vi "Owning System.vi"(8 "error in (no error)":errorcluster, 11 "Group in":refnum<class "Group.lvclass">) -> (0 "error out":errorcluster, 2 "Owning System":string, 3 "Group out":refnum<class "Group.lvclass">)   [LabVIEW 2020, in "VolatusConfig.lvlib" / "Group.lvclass"]
uses:
  Group.lvclass
  Group.lvclass/Group.ctl
  lv-cdm/CDM-Config/Config Manager/Config Manager.lvclass
  VolatusConfig.lvlib
  Meta Type.ctl
  lv-cdm/CDM-Config/Config Element/Config Element.lvclass
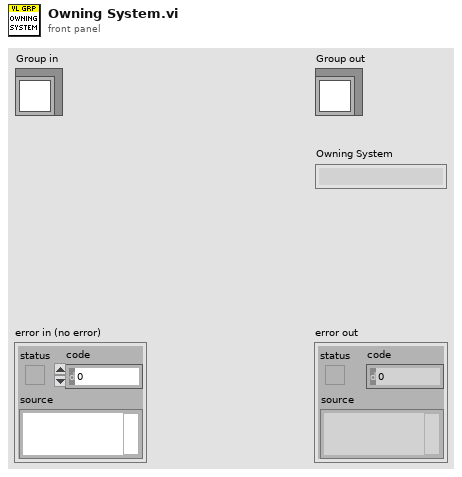
[diagram p1: front panel]
types:
  T1 = typedef "VolatusConfig.lvlib/Meta Type.ctl" = enum16{"VL_System", "VL_Cluster", "VL_Node", "VL_Task", "VL_Group", "VL_Channel", "VL_Task_List"}
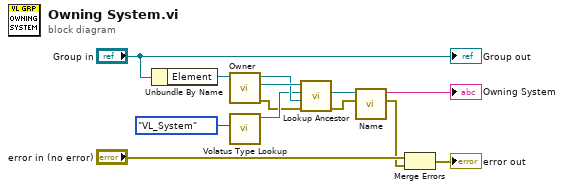
[diagram p0: block diagram]
diagram:
  n1 = Unbundle By Name("Group in") -> ("Element"=w11:refnum<class "Config Element.lvclass">)
  n2 = call "Owner.vi"("Config Element in"=w11) -> ("error out"=w3:errorcluster, "Owner"=w10:refnum<class "Config Manager.lvclass">, "Config Element out"=w9:refnum<class "Config Element.lvclass">)  [unwired: 8 in]
  n3 = call "Volatus Type Lookup.vi"("Meta Type"=Meta_Type."VL_System") -> ("Config Lookup out"=w7:refnum<class "Config Lookup.lvclass">)  [unwired: 9 in, 1 out]
  n4 = call "Lookup Ancestor.vi"("error in (no error)"=w3, "Descendant"=w9, "Lookup"=w7, "Config Manager in"=w10) -> ("error out"=w2:errorcluster, "Ancestor"=w6:refnum<class "Config Element.lvclass">)  [unwired: 5 in, 1 out]
  n5 = call "Name.vi"("error in (no error)"=w2, "Config Element in"=w6) -> ("error out"=w1:errorcluster, "Name"=→"Owning System":string)  [unwired: 8 in]
  n6 = Merge Errors("error in (no error)", w1) -> (→"error out":errorcluster)
  "Group out" <- "Group in"
